vi "Channel Value Retention Service Main.vi"() -> ()   [LabVIEW 2015]
uses:
  NationalInstruments.VeriStand.SystemStorageUI
  NationalInstruments.VeriStand.SystemStorage
  <vilib>/NI Veristand/Execution/Workspace/WorkspaceAPI.ctl
  <vilib>/NI Veristand/Execution/Workspace/NI VeriStand - Get Multiple Channel Values.vi
  <vilib>/NI Veristand/Execution/Workspace/NI_VS Workspace ExecutionAPI.lvlib
  <vilib>/NI Veristand/Custom Device Tools/Custom Device Utility Library/Custom Device Utility Library.lvlib
  NationalInstruments.VeriStand.ClientAPI
panel:
  in  "NIVS.System Definition Root":refnum<k24>
  in  "Tree Browser":refnum<k24>(container)
  in  "NIVS.Project File Path":path
  in  "Single Node Browser":refnum<k24>(container)
  in  "NIVS.Workspace Event":refnum<event-registration>
  in  "NIVS.INI File Path":path
  in  "NIVS.Gateway IP Address":string
  in  "Configure":bool
  in  "Current Channels Monitored":i32(listbox)
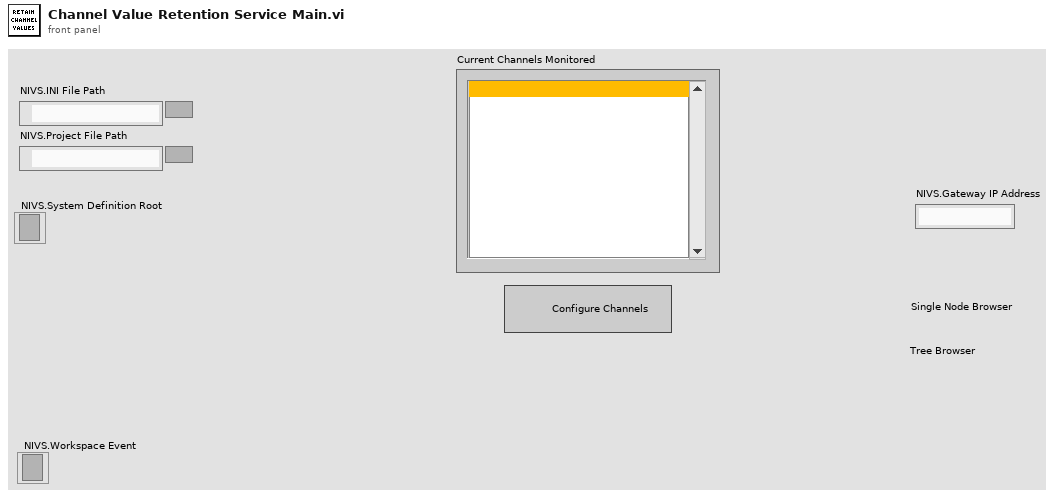
[diagram p1: front panel]
types:
  T1 = typedef "NI_VS Workspace ExecutionAPI.lvlib/WorkspaceAPI.ctl" = refnum<k24>
  T2 = cluster{"SDF path":path, "WorkspaceManager":T1, "Channels":string[], "Values":dbl[]}
  T3 = typedef "NI_VS Workspace ExecutionAPI.lvlib/SystemStateEventRef.ctl" = cluster{"CustDatRef":refnum<user-event>, "EvtRef":refnum<k27>, "Target State User Event":refnum<user-event>}
  T4 = typedef "NI_VS Workspace ExecutionAPI.lvlib/SystemStateRegEventRef.ctl" = refnum<event-registration>
  T5 = enum32{"Invalid", "Standard", "Closed", "Hidden", "Minimized", "Maximized"}
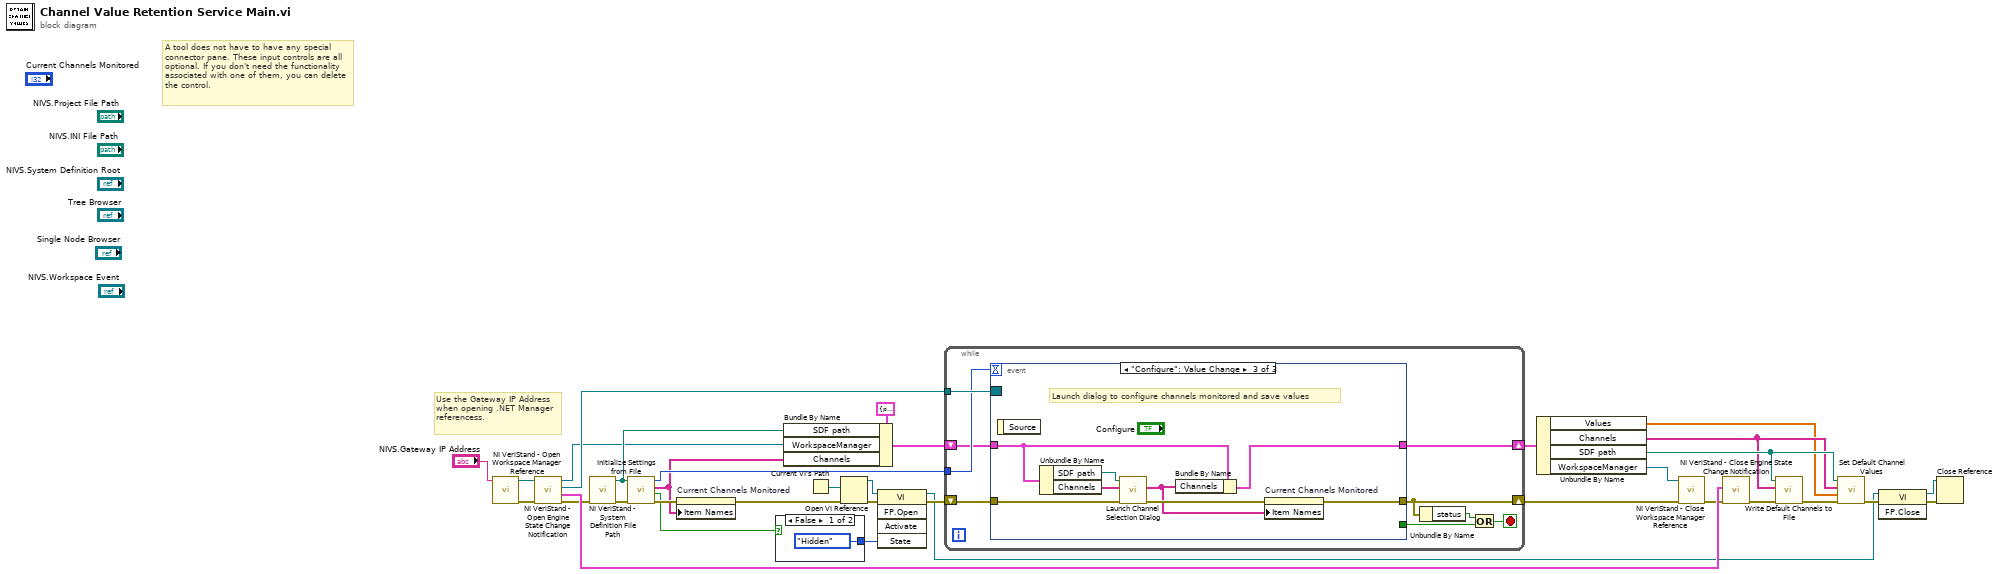
[diagram p0: block diagram]
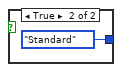
[diagram p2: hidden frame]
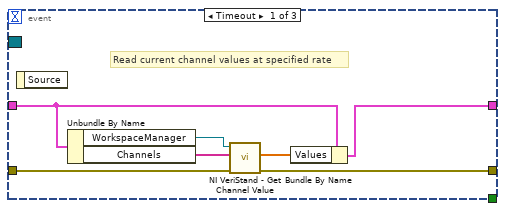
[diagram p3: hidden frame]
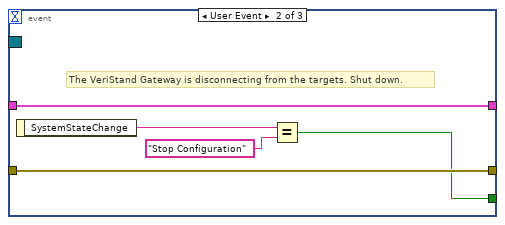
[diagram p4: hidden frame]
diagram:
  # "Use the Gateway IP Address when opening .NET Manager referencess."
  # "A tool does not have to have any special connector pane. These input controls are all optional. If you don't need the functionality associated with one of them, you can delete the control."
  n1 = call <vilib>:"NI VeriStand - Open Workspace Manager Reference.vi"("Gateway IP Address (\"\": localhost)"="NIVS.Gateway IP Address") -> ("error out"=w33:errorcluster, "WorkspaceManager"=w34:T1)  [unwired: 9 in]
  n2 = call <vilib>:"NI VeriStand - Open Engine State Change Notification.vi"("error in (no error)"=w33, "WorkspaceManager in"=w34) -> ("error out"=w27:errorcluster, "SystemStateRefs"=w30:T3, "SystemChangeEventRef"=w31:T4, "WorkspaceManager out"=w11:T1)  [unwired: 6 in]
  n3 = call <vilib>:"NI VeriStand - System Definition File Path.vi"("error in (no error)"=w27) -> ("error out"=w20:errorcluster, "SDF path"=w12:path)  [unwired: 9 in]
  n4 = call "Initialize Settings from File.vi"("error in (no error)"=w20, "SDF Path"=w12) -> ("error out"=w29:errorcluster, "Visible?"=w19:bool, "Channels"=w10:string[], "Rate"=w28:i32)  [unwired: 6 in]
  n5 = property on="Current Channels Monitored" class="LstBox (strict)"(error in=w29, "Item Names"=w10) -> (error out=w25:errorcluster)  [unwired: 1 in, 1 out]
  n6 = case shown="False" w19 {
    tunnel: [T5."Hidden" ("State") T5."Standard" ("State")] -> w22
    frame False {
    }
    frame True {
    }
  }
  n7 = Bundle By Name(cluster=T2 {"SDF path"=path "", "WorkspaceManager"=refnum, "Channels"=[], "Values"=[]}, "SDF path"=w12, "WorkspaceManager"=w11, "Channels"=w10) -> (w9:T2)
  n8 = Current VI's Path() -> (path=w26:path)
  n9 = Open VI Reference(vi path=w26, error in (no error)=w25) -> (vi reference=w24:refnum<vi>, error out=w23:errorcluster)  [unwired: 4 in]
  n10 = invoke class="VI" method="FP.Open"(reference=w24, error in=w23, "State"=w22) -> (reference out=w1:refnum<vi>, error out=w21:errorcluster)  [unwired: 2 in, 3 out]
  n11 = while {
    shift-right: [w41] -> w16
    shift-left: w21 -> [w43]
    tunnel: w31 -> [w45]
    tunnel: w28 -> [w39]
    shift-right: [w37] -> w8
    shift-left: w9 -> [w38]
    stop <- w44 stop-if-true
    n12 = event shown="[2] \"Configure\": Value Change" {
      selector: w45 -> [_ _ _]
      dyn-events: _ -> [_ _ _]
      timeout: w39 -> [_ _ _]
      tunnel: [_ w53 _] -> w40
      tunnel: w43 -> [w52 w55 w64]
      tunnel: [w51 w55 w65] -> w41
      tunnel: w38 -> [w48 w54 w58]
      tunnel: [w46 w54 w59] -> w37
      event Timeout {
        # "Read current channel values at specified rate"
        n13 = event-data() -> ()  [unwired: 1 in, 1 out]
        n14 = Unbundle By Name(w48) -> ("WorkspaceManager"=w50:T1, "Channels"=w49:string[])
        n15 = call-poly <vilib>:"NI VeriStand - Get Channel Value.vi"("error in (no error)"=w52, "Channels"=w49, "WorkspaceManager in"=w50) -> ("error out"=w51:errorcluster, "Values"=w47:dbl[])  [unwired: 6 in, 1 out]
        n16 = Bundle By Name(cluster=w48, "Values"=w47) -> (w46:T2)
      }
      event User Event {
        # "The VeriStand Gateway is disconnecting from the targets. Shut down."
        n17 = event-data() -> ("SystemStateChange"=w57:string)  [unwired: 1 in]
        n18 = Equal?(x=w57, y="Stop Configuration") -> (x = y?=w53:bool)
      }
      event "Configure": Value Change {
        # "Launch dialog to configure channels monitored and save values"
        n19 = event-data() -> ()  [unwired: 1 in, 1 out]
        n20 = Unbundle By Name(w58) -> ("SDF path"=w62:path, "Channels"=w61:string[])
        n21 = call "Launch Channel Selection Dialog.vi"("error in (no error)"=w64, "Channels to Highlight"=w61, "SDF Path"=w62) -> ("error out"=w63:errorcluster, "Channels Selected"=w60:string[])  [unwired: 6 in, 1 out]
        n22 = Bundle By Name(cluster=w58, "Channels"=w60) -> (w59:T2)
        n23 = property on="Current Channels Monitored" class="LstBox (strict)"(error in=w63, "Item Names"=w60) -> (error out=w65:errorcluster)  [unwired: 1 in, 1 out]
      }
    }
    n24 = Unbundle By Name(w41) -> ("status"=w42:bool)
    n25 = Or(x=w42, y=w40) -> (x .or. y?=w44:bool)
  }
  n26 = Unbundle By Name(w8) -> ("Values"=w4:dbl[], "Channels"=w5:string[], "SDF path"=w6:path, "WorkspaceManager"=w7:T1)
  n27 = call <vilib>:"NI VeriStand - Close Workspace Manager Reference.vi"("error in (no error)"=w16, "WorkspaceManager"=w7) -> ("error out"=w17:errorcluster)  [unwired: 9 in]
  n28 = call <vilib>:"NI VeriStand - Close Engine State Change Notification.vi"("error in (no error)"=w17, "SystemStateRefs"=w30) -> ("error out"=w18:errorcluster)  [unwired: 9 in]
  n29 = call "Write Default Channels to File.vi"("error in (no error)"=w18, "Channels"=w5, "SysDef File Path"=w6) -> ("error out"=w15:errorcluster)  [unwired: 8 in]
  n30 = call "Set Default Channel Values.vi"("error in (no error)"=w15, "Values"=w4, "Channels"=w5, "SysDef Path"=w6) -> ("error out"=w14:errorcluster)  [unwired: 7 in]
  n31 = invoke class="VI" method="FP.Close"(reference=w1, error in=w14) -> (reference out=w2:refnum<vi>, error out=w3:errorcluster)  [unwired: 1 in, 1 out]
  n32 = Close Reference(reference=w2, error in (no error)=w3) -> ()  [unwired: 1 out]
